vi "test_libssh2_version.vi"() -> ()   [LabVIEW 2017, in "unit_tests.lvlib"]
uses:
  unit_tests.lvlib
  libssh2/libssh2_init_default.vi
  <vilib>/regexp/Match Regular Expression.xnode
  libssh2/libssh2.lvlib
  <vilib>/PNR/Transparent Assertions/Transparent Assertions/Transparent Assertions.lvlib
panel:
  out "error out":errorcluster
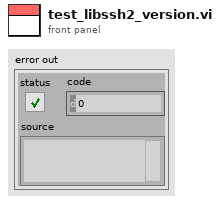
[diagram p1: front panel]
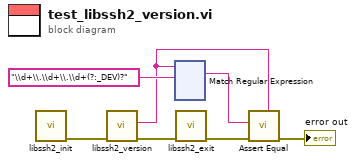
[diagram p0: block diagram]
diagram:
  n1 = call-poly "libssh2_init.vi"() -> ("error out"=w7:errorcluster)  [unwired: 11 in]
  n2 = call "libssh2_version.vi"("error in (no error)"=w7) -> ("error out"=w6:errorcluster, "version"=w1:string)  [unwired: 9 in]
  n3 = xnode "Match Regular Expression"("input string"=w1, "regular expression"="\\d+\\.\\d+\\.\\d+(?:_DEV)?") -> ("whole match"=w2:string)  [unwired: 4 in, 4 out]
  n4 = call "libssh2_exit.vi"("error in (no error)"=w6) -> ("error out"=w4:errorcluster)  [unwired: 10 in]
  n5 = call <vilib>:"Assert Equal.vi"("Expected"=w1, "error in (no error)"=w4, "Actual"=w2) -> ("error out"=→"error out":errorcluster)  [unwired: 8 in]
